vi "Pie Chart Test.vi"() -> ()   [LabVIEW 2020]
uses:
  Pie Chart/Pie Chart.xctl
panel:
  out "Pie Chart":T1(xcontrol)
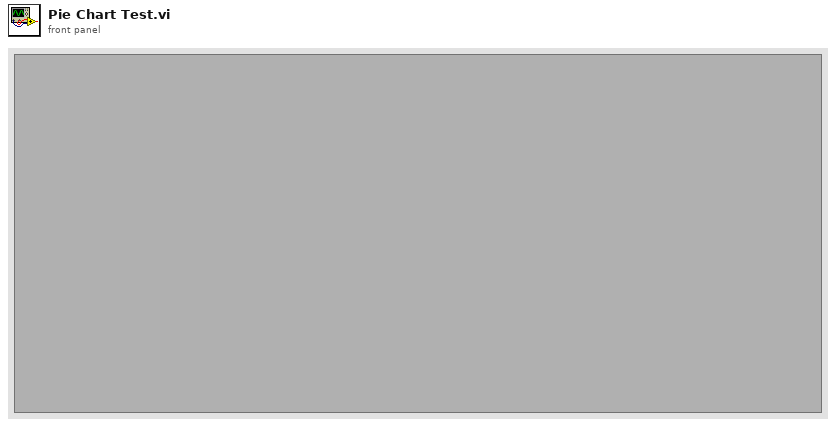
[diagram p1: front panel]
types:
  T1 = cluster{"Plot Title":string, "Plots":cluster{"Name":string, "Value":dbl, "Color":u32}[]}
  T2 = cluster{"Plot Title":string, "Plots":cluster{"Name":string, "Value":dbl, u32}[]}
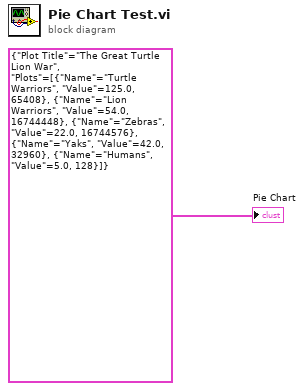
[diagram p0: block diagram]
diagram:
  "Pie Chart" <- T2 {"Plot Title"="The Great Turtle Lion War", "Plots"=[{"Name"="Turtle Warriors", "Value"=125.0, 65408}, {"Name"="Lion Warriors", "Value"=54.0, 16744448}, {"Name"="Zebras", "Value"=22.0, 16744576}, {"Name"="Yaks", "Value"=42.0, 32960}, {"Name"="Humans", "Value"=5.0, 128}]} ("Pie Chart")
